vi "measure_amplitude.vi"(8 "error in":errorcluster, 11 "Coarse Approach in":refnum<class "Coarse Approach.lvclass">) -> (0 "error out":errorcluster, 1 "Amplitude stdev":dbl, 2 "Amplitude mean":dbl, 3 "Coarse Approach out":refnum<class "Coarse Approach.lvclass">)   [LabVIEW 2020, in "Coarse Approach.lvclass"]
uses:
  Coarse Approach.lvclass
  Coarse Approach.lvclass/Coarse Approach.ctl
  Lock-In Amplifier/Lock-In Amplifier.lvclass
  <vilib>/Analysis/NI_AALBase.lvlib
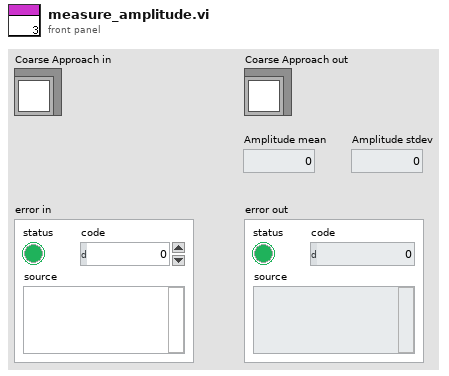
[diagram p1: front panel]
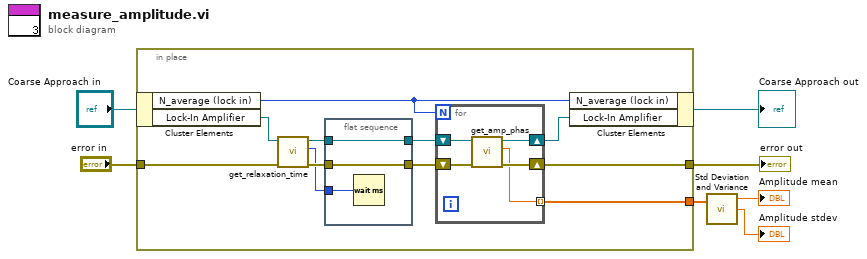
[diagram p0: block diagram]
diagram:
  n1 = in-place {
    in-place-border: "error in" -> [w17]
    in-place-border: [w10] -> w5
    in-place-border: [w9] -> w3
    n2 = in-place-cluster #1("Coarse Approach in") -> ("N_average (lock in)"=w8:i32, "Lock-In Amplifier"=w18:refnum<class "Lock-In Amplifier.lvclass">)
    n3 = call "get_relaxation_time.vi"("error in"=w17, "Lock-In Amplifier"=w18) -> ("error out"=w15:errorcluster, "Wait time (ms)"=w14:u32, "Lock-In Amplifier"=w16:refnum<class "Lock-In Amplifier.lvclass">)  [unwired: 7 in]
    n4 = flat-sequence {
      tunnel: [w26] -> w13
      tunnel: w16 -> [w26]
      tunnel: [w25] -> w12
      tunnel: w15 -> [w25]
      tunnel: w14 -> [w24]
      frame #0 {
        n5 = Wait (ms)(milliseconds to wait=w24) -> ()  [unwired: 1 out]
      }
    }
    n6 = for {
      N: w8 -> [_]
      tunnel: [w19] -> w9 mode=indexing
      shift-right: [w21] -> w11
      shift-left: w13 -> [w23]
      shift-right: [w20] -> w10
      shift-left: w12 -> [w22]
      n7 = call-dynamic "get_amp_phas.vi"("error in (no error)"=w22, "Lock-In Amplifier in"=w23) -> ("error out"=w20:errorcluster, "Amplitude (V rms)"=w19:dbl, "Lock-In Amplifier out"=w21:refnum<class "Lock-In Amplifier.lvclass">)  [unwired: 6 in, 1 out]
    }
    n8 = in-place-cluster #1("N_average (lock in)"=w8, "Lock-In Amplifier"=w11) -> (→"Coarse Approach out":refnum<class "Coarse Approach.lvclass">)
  }
  "error out" <- w5
  n9 = call <vilib>:"Std Deviation and Variance.vi"("X"=w3) -> ("mean"=→"Amplitude mean":dbl, "standard deviation"=→"Amplitude stdev":dbl)  [unwired: 1 in, 1 out]
